vi "INTELLIFAUCET Need Adjustment PID.vi"(0 "Previous MicroAmp":i32, 1 "GPM reading":dbl, 3 "Use Proportion Valve":bool, 4 "GPM Target(3)":dbl, 5 "Error In":errorcluster, 6 "Use Fuzzy Logic":bool, 7 "ErrorPassBand(%)":dbl=0.01, 8 "Elapsed Time (sec)":dbl, 9 "State":T2, 10 "PID gains":T3={"proportional gain (Kc)"=0.1, "integral time (Ti, min)"=0.01, "derivative time (Td, min)"=0.0} {"derivative time (Td, min)" format="%.3f"; "integral time (Ti, min)" format="%.3f"; "proportional gain (Kc)" format="%.3f"}, 11 "K(0.1)":dbl=0.1, 12 "TEMP,FLOW":T1=enum."FLOW", 13 "output range":cluster{"output high":dbl, "output low":dbl}={"output high"=140.0, "output low"=40.0} {"output low" format="%.2f"; "output high" format="%.2f"}) -> (14 "Going into Correction Loop?":bool, 15 "Adjustment Factor":dbl, 17 "Control Variable (Temp/GPM) Output":dbl, 18 "Micro Amp":i32, 19 "Error Out":errorcluster)   [LabVIEW 2016]
uses:
  Type Definitions/HEWH Purge Draw.ctl
  Type Definitions/INTELLIFAUCT Temp Flow.ctl
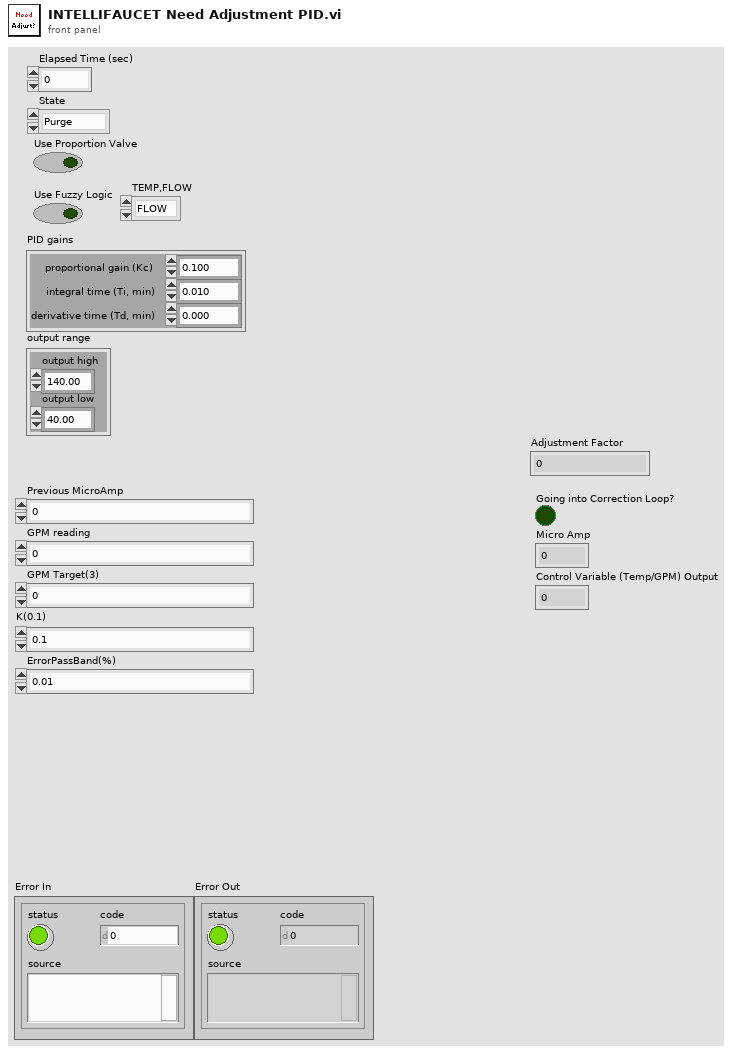
[diagram p1: front panel]
types:
  T1 = typedef "INTELLIFAUCT Temp Flow.ctl" = enum8{"TEMP", "FLOW"}
  T2 = typedef "HEWH Purge Draw.ctl" = enum16{"Purge", "Draw"}
  T3 = cluster{"proportional gain (Kc)":dbl, "integral time (Ti, min)":dbl, "derivative time (Td, min)":dbl}
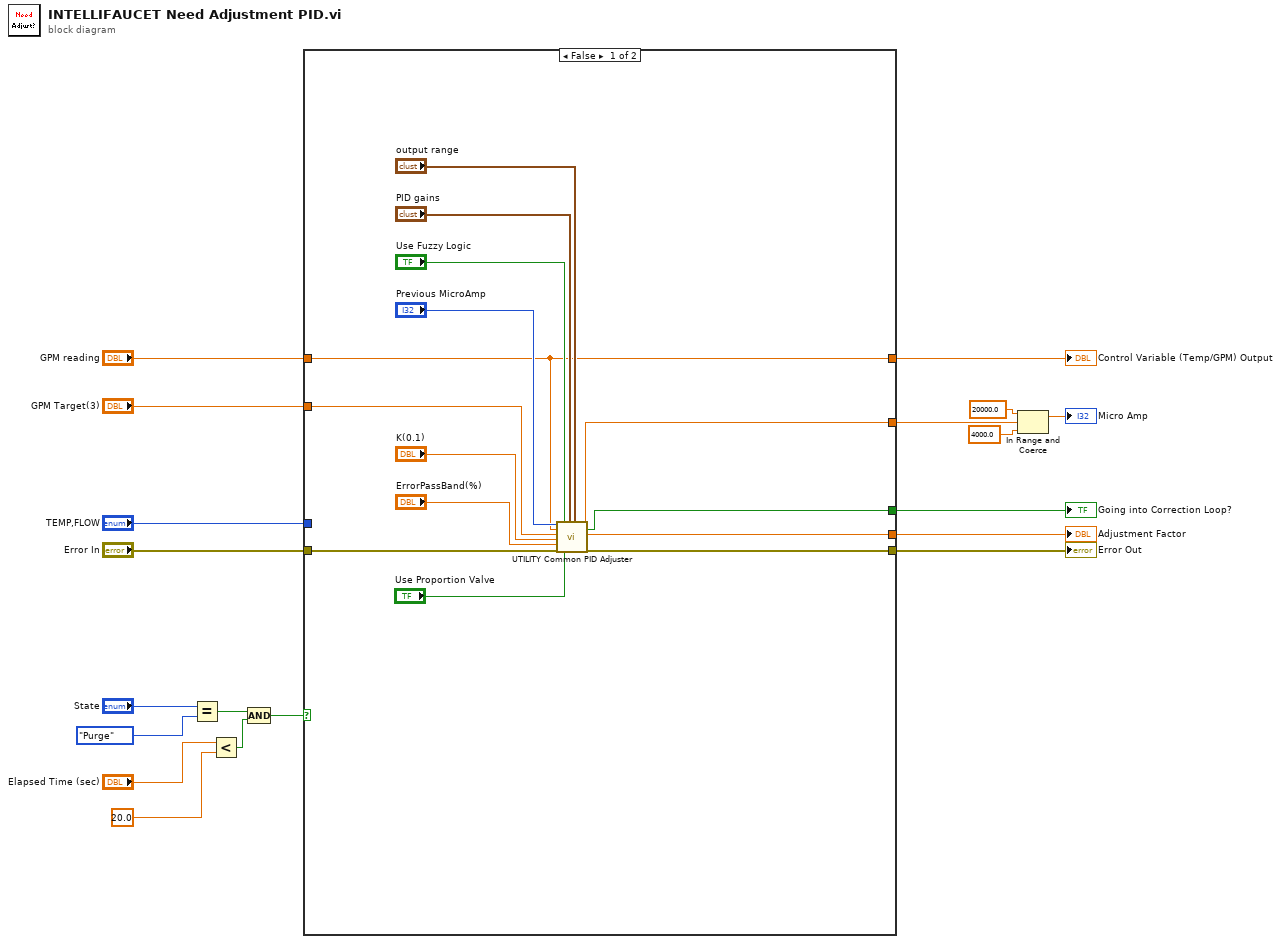
[diagram p0: block diagram]
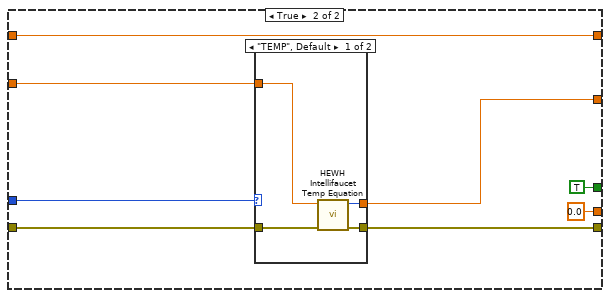
[diagram p2: hidden frame]
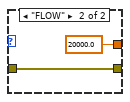
[diagram p3: hidden frame]
diagram:
  n1 = Equal?(x="State", y=HEWH_Purge_Draw."Purge") -> (x = y?=w14:bool)
  n2 = Less?(x="Elapsed Time (sec)", y=20.0) -> (x < y?=w11:bool)
  n3 = Compound Arithmetic op=AND(w14, w11) -> (w10:bool)
  n4 = case shown="False" w10 {
    tunnel: [w26 w36] -> w9
    tunnel: [w25 0.0 ("Adjustment Factor")] -> w8
    tunnel: [w24 TRUE ("Going into Correction Loop?")] -> w7
    tunnel: [w23 w38] -> w6
    tunnel: [w22 w41] -> w5
    tunnel: "GPM reading" -> [w22 w41]
    tunnel: "Error In" -> [w21 w37]
    tunnel: "TEMP,FLOW" -> [_ w35]
    tunnel: "GPM Target(3)" -> [w20 w34]
    frame False {
      n5 = call "UTILITY Common PID Adjuster.vi"("Previous Value"="Previous MicroAmp", "Current Rate"=w22, "Scan Rate Target"=w20, "K(7) - Adjustment Factor"="K(0.1)", "ErrorPassBand(%)"="ErrorPassBand(%)", "Error In"=w21, "Use Fuzzy Logic"="Use Fuzzy Logic", "Use Proportion Valve"="Use Proportion Valve", "PID gains"="PID gains", "output range"="output range") -> ("New MicroAmp"=w23:dbl, "Going into Correction Loop?"=w24:bool, "Adjustment Factor"=w25:dbl, "Error Out"=w26:errorcluster)  [unwired: 6 in]
    }
    frame True {
      n6 = case shown="\"TEMP\", Default" w35 {
        tunnel: [w45 20000.0 ("upper limit")] -> w38
        tunnel: w37 -> [w44 w46]
        tunnel: [w43 w46] -> w36
        tunnel: w34 -> [w42 _]
        frame "TEMP", Default {
          n7 = call "HEWH Intellifaucet Temp Equation.vi"("Error In"=w44, "Temp/GPM Target"=w42) -> ("Error Out"=w43:errorcluster, "Temp uA"=w45:i32)  [unwired: 8 in]
        }
        frame "FLOW" {
        }
      }
    }
  }
  "Error Out" <- w9
  "Going into Correction Loop?" <- w7
  "Control Variable (Temp/GPM) Output" <- w5
  "Adjustment Factor" <- w8
  n8 = In Range and Coerce(upper limit=20000.0, x=w6, lower limit=4000.0) -> (coerced(x)=→"Micro Amp":dbl)  [unwired: 1 out]
